vi "VarMan_Register_Computer.vi"() -> ()   [LabVIEW 2020]
uses:
  <resource>/logosbrw.dll
panel:
  in  "Machine Name or IP Address":string
  in  "Cancel":bool
  in  "OK":bool
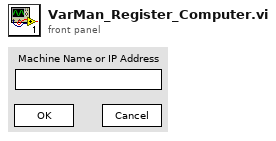
[diagram p1: front panel]
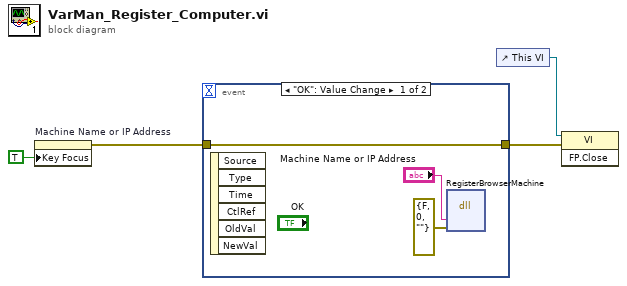
[diagram p0: block diagram]
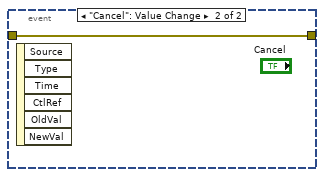
[diagram p2: hidden frame]
diagram:
  n1 = property on="Machine Name or IP Address" class="Str"("Key Focus"=TRUE) -> (error out=w3:errorcluster)  [unwired: 2 in, 1 out]
  n2 = event shown="[0] \"OK\": Value Change" {
    selector: _ -> [_ _]
    dyn-events: _ -> [_ _]
    timeout: _ -> [_ _]
    tunnel: w3 -> [w7 w8]
    tunnel: [w7 w8] -> w1
    event "OK": Value Change {
      n3 = event-data() -> ()  [unwired: 1 in, 6 out]
      n4 = dll-call lib="e:/builds/penguin/labview/branches/2020/dev/dist/resource/logosbrw.dll" fn="RegisterBrowserMachine"("machine"="Machine Name or IP Address", "err"=errorcluster {"status"=FALSE, "code"=0, "source"=""} ("error in (no error)")) -> ()  [unwired: 6 in, 2 out]
    }
    event "Cancel": Value Change {
      n5 = event-data() -> ()  [unwired: 1 in, 6 out]
    }
  }
  n6 = control-ref of="This VI"() -> (w2:refnum<vi>)
  n7 = invoke class="VI" method="FP.Close"(reference=w2, error in=w1) -> ()  [unwired: 1 in, 3 out]
